vi "Update Server Start Async.vi"(8 "error in (no error)":errorcluster, 11 "Server class in":refnum<vi>) -> (0 "error out":errorcluster, 3 "Server class out":refnum<vi>)   [LabVIEW 2019, in "gRPC Template Creation Utility.lvlib"]
uses:
  gRPC Template Creation Utility.lvlib
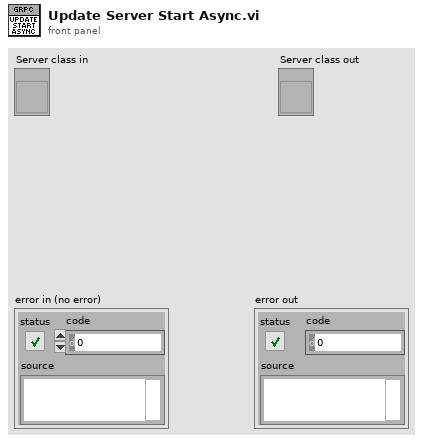
[diagram p1: front panel]
types:
  T1 = typedef "LVPointTypeDef.ctl" = cluster{"Horizontal":i16, "Vertical":i16}
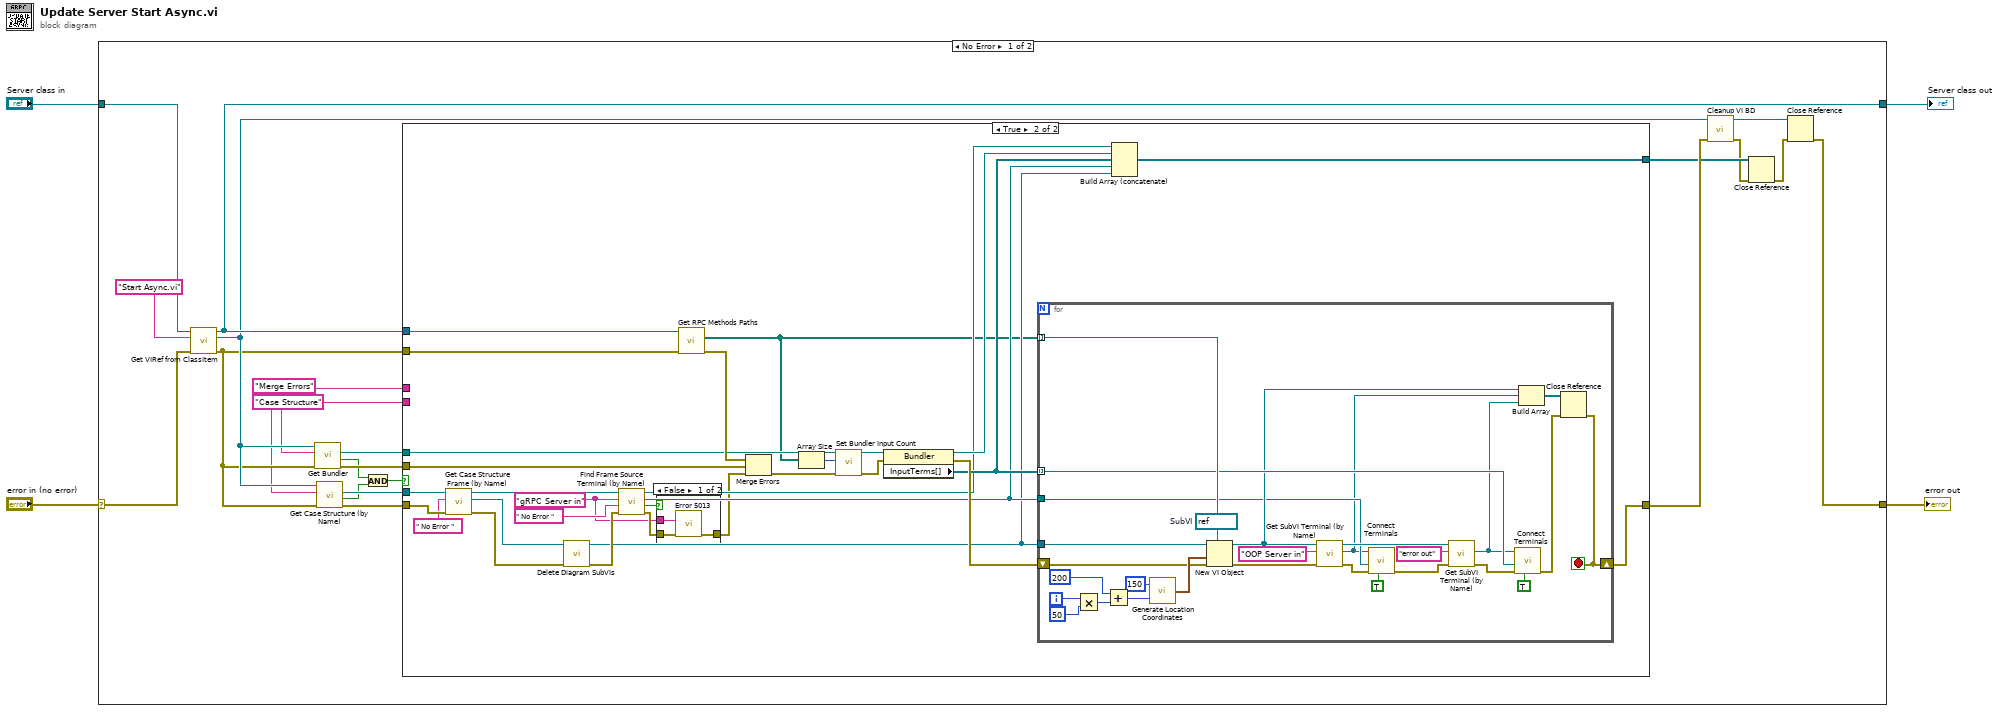
[diagram p0: block diagram]
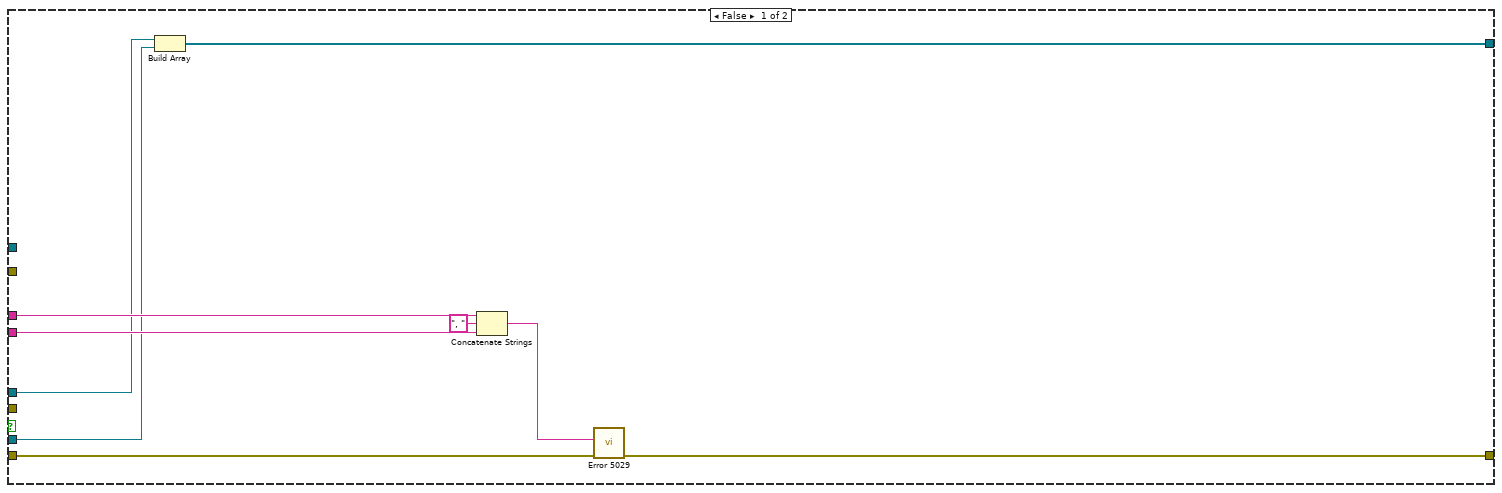
[diagram p2: hidden frame]
diagram:
  n1 = case shown="No Error" "error in (no error)" {
    selector: "error in (no error)" -> [w23 w98]
    tunnel: "Server class in" -> [w24 w97]
    tunnel: [w10 w98] -> w2
    tunnel: [w20 w97] -> w1
    frame No Error {
      w5 = "Merge Errors" ("Label")
      w6 = "Case Structure" ("y")
      n2 = call "Get VIRef from ClassItem.vi"("error in (no error)"=w23, "Item Name"="Start Async.vi", "LVClassLibrary in"=w24) -> ("error out"=w17:errorcluster, "VIref out"=w18:refnum<vi>, "LVClassLibrary out"=w20:refnum<vi>)  [unwired: 5 in, 1 out]
      n3 = call "Get Bundler.vi"("error in (no error)"=w17, "Label"=w5, "Owner VI in"=w18) -> ("error out"=w16:errorcluster, "Found ?"=w9:bool, "Bundler ref out"=w15:refnum<vi>)  [unwired: 5 in, 1 out]
      n4 = call "Get Case Structure (by Name).vi"("error in (no error)"=w17, "Case Structure name"=w6, "VI ref in"=w18) -> ("error out"=w21:errorcluster, "Found ?"=w8:bool, "CaseStructure out"=w22:refnum<vi>)  [unwired: 5 in, 1 out]
      n5 = And(x=w9, y=w8) -> (x .and. y?=w7:bool)
      n6 = case shown="True" w7 {
        tunnel: w22 -> [w27 w64]
        tunnel: w21 -> [w34 w63]
        tunnel: w20 -> [_ w59]
        tunnel: [w33 w57] -> w19
        tunnel: w17 -> [_ w56]
        tunnel: w16 -> [_ w52]
        tunnel: w15 -> [w28 w50]
        tunnel: [w26 w40] -> w13
        tunnel: w6 -> [w30 _]
        tunnel: w5 -> [w32 _]
        frame False {
          n7 = Build Array(w28, w27) -> (w26:refnum<vi>[])
          n8 = Concatenate Strings(w32, ", " ("string"), w30) -> (w29:string)
          n9 = call "Error 5029.vi"("error in (no error)"=w34, "Element Name"=w29) -> ("error out"=w33:errorcluster)  [unwired: 9 in]
        }
        frame True {
          w36 = "gRPC Server in" ("element")
          n10 = call "Get Case Structure Frame (by Name).vi"("error in (no error)"=w63, "element"=" No Error ", "CaseStructure in"=w64) -> ("error out"=w61:errorcluster, "Frame ref out"=w60:refnum<vi>, "CaseStructure out"=w55:refnum<vi>)  [unwired: 5 in, 1 out]
          n11 = call "Delete Diagram SubVIs.vi"("error in (no error)"=w61, "Diagram in"=w60) -> ("error out"=w54:errorcluster, "Diagram out"=w41:refnum<vi>)  [unwired: 8 in]
          n12 = call "Find Frame Source Terminal (by Name).vi"("error in (no error)"=w54, "Frame Name"=" No Error " ("element"), "Terminal Name"=w36, "CaseStructure in"=w55) -> ("error IO"=w37:errorcluster, "Found ?"=w38:bool, "Terminal ref"=w43:refnum<vi>, "CaseStructure out"=w42:refnum<vi>)  [unwired: 4 in]
          n13 = case shown="False" w38 {
            tunnel: w37 -> [w67 w68]
            tunnel: w36 -> [w66 _]
            tunnel: [w65 w68] -> w35
            frame False {
              n14 = call "Error 5013.vi"("error in (no error)"=w67, "Element Name"=w66) -> ("error out"=w65:errorcluster)  [unwired: 9 in]
            }
            frame True {
            }
          }
          n15 = call "Get RPC Methods Paths.vi"("error in (no error)"=w56, "LVClassLibrary in"=w59) -> ("error out"=w53:errorcluster, "RPC Method Paths"=w39:path[])  [unwired: 6 in, 2 out]
          n16 = Merge Errors(w53, w52, w35) -> (w49:errorcluster)
          n17 = Array Size(array=w39) -> (size(s)=w48:i32)
          n18 = call "Set Bundler Input Count.vi"("error in (no error)"=w49, "Numeric"=w48, "Bundler in"=w50) -> ("error out"=w46:errorcluster, "Bundler out"=w47:refnum<vi>)  [unwired: 7 in]
          n19 = property class="Bundler"(reference=w47, error in=w46) -> (reference out=w44:refnum<vi>, error out=w51:errorcluster, "InputTerms[]"=w45:refnum<vi>[])
          n20 = for {
            tunnel: w41 -> [w89]
            tunnel: w39 -> [w87] mode=indexing
            tunnel: w43 -> [w74]
            shift-right: [w69] -> w57
            shift-left: w51 -> [w86]
            tunnel: w45 -> [w77] mode=indexing
            i -> [w88]
            stop <- w69 stop-if-true
            w90 = refnum<vi> refnum  # SubVI
            n21 = Multiply(x=w88, y=50) -> (x*y=w94:i32)
            n22 = Add(x=i16 200 ("Horizontal"), y=w94) -> (x+y=w95:i32)
            n23 = call "Generate Location Coordinates.vi"("Vertical"=w95, "Horizontal"=i16 150) -> ("Location out"=w96:T1)
            n24 = New VI Object(vi object class=w90, owner refnum=w89, position/next to=w96, 6:w87, 8:w86) -> (object refnum=w75:refnum<vi>, 0:w83:errorcluster)  [unwired: 3 in]
            n25 = call "Get SubVI Terminal (by Name).vi"("error in (no error)"=w83, "Terminal name"="OOP Server in", "SubVI in"=w75) -> ("error out"=w84:errorcluster, "SubVI Term ref"=w71:refnum<vi>, "SubVI out"=w79:refnum<vi>)  [unwired: 5 in, 1 out]
            n26 = call "Connect Terminals.vi"("Auto Route? (F)"=TRUE, "Error In"=w84, "Source Terminal"=w74, "Sink Terminal"=w71) -> ("Error Out"=w81:errorcluster)  [unwired: 7 in]
            n27 = call "Get SubVI Terminal (by Name).vi"("error in (no error)"=w81, "Terminal name"="error out", "SubVI in"=w79) -> ("error out"=w78:errorcluster, "SubVI Term ref"=w70:refnum<vi>)  [unwired: 5 in, 2 out]
            n28 = call "Connect Terminals.vi"("Auto Route? (F)"=TRUE, "Error In"=w78, "Source Terminal"=w77, "Sink Terminal"=w70) -> ("Error Out"=w72:errorcluster)  [unwired: 7 in]
            n29 = Build Array(w75, w71, w70) -> (w73:refnum<vi>[])
            n30 = Close Reference(reference=w73, error in (no error)=w72) -> (error out=w69:errorcluster)
          }
          n31 = Build Array (concatenate)(w42, w44, w45, w43, w41) -> (w40:refnum<vi>[])
        }
      }
      n32 = call "Cleanup VI BD.vi"("error in (no error)"=w19, "VI in"=w18) -> ("error out"=w12:errorcluster, "VI out"=w14:refnum<vi>)  [unwired: 8 in]
      n33 = Close Reference(reference=w13, error in (no error)=w12) -> (error out=w11:errorcluster)
      n34 = Close Reference(reference=w14, error in (no error)=w11) -> (error out=w10:errorcluster)
    }
    frame Error {
    }
  }
  "error out" <- w2
  "Server class out" <- w1
